vi "ListSelectedValue.vi"(8 "Language":u32, 9 "值表数组":string[][](array[string]), 10 "已选信号列表":string[][](array[string])) -> (3 "SelectList":string(tree))   [LabVIEW 2015]
panel:
  out "txtTitle":string
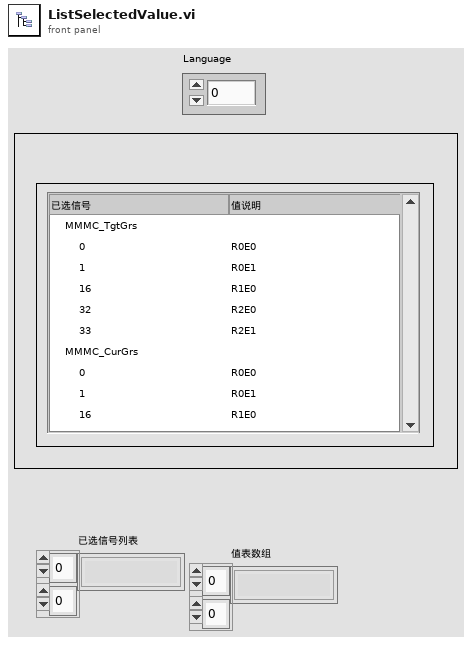
[diagram p1: front panel]
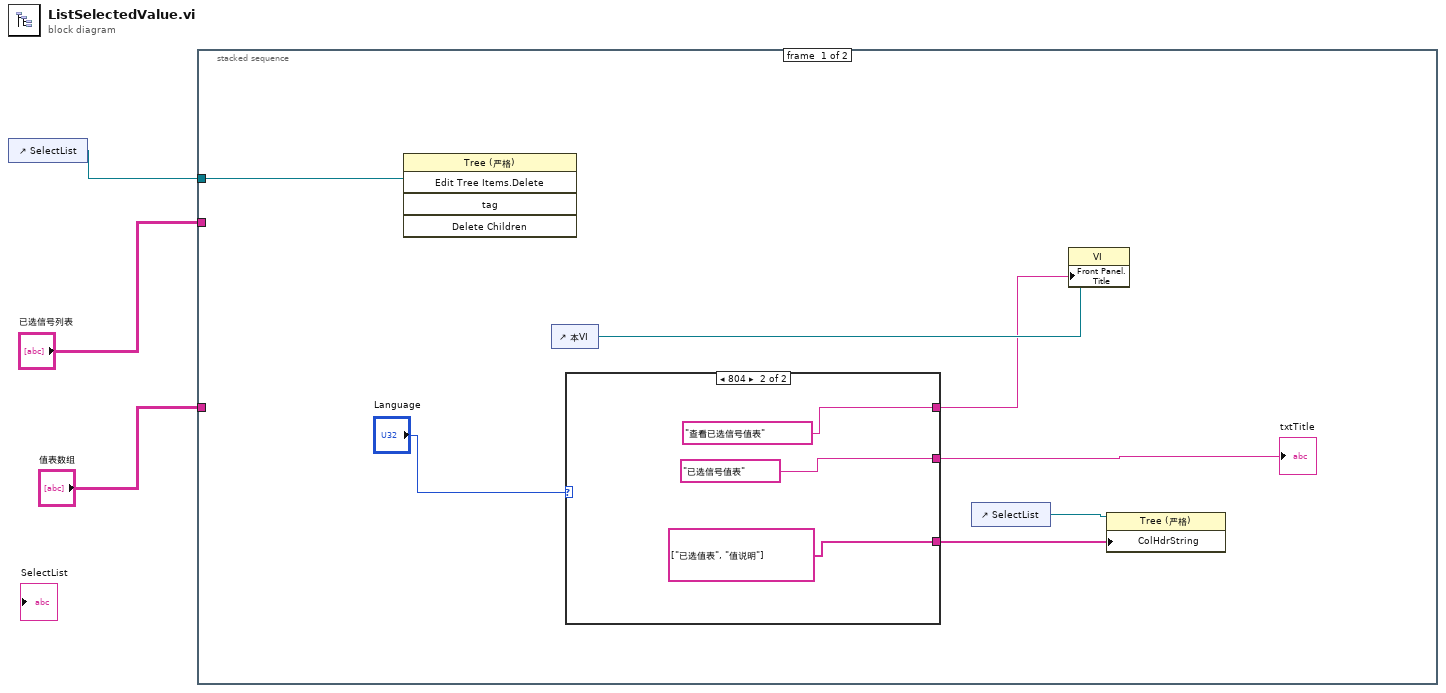
[diagram p0: block diagram]
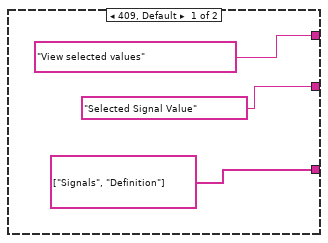
[diagram p2: hidden frame]
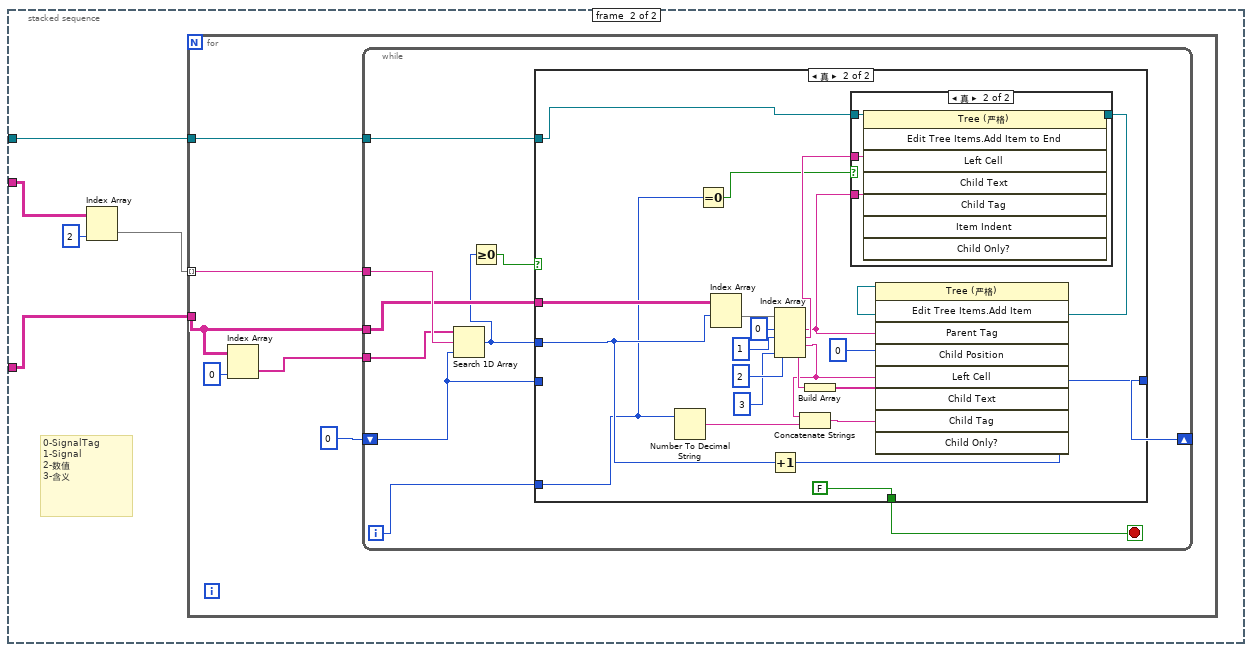
[diagram p3: hidden frame]
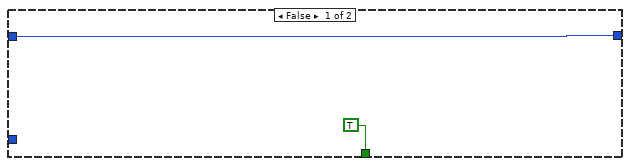
[diagram p4: hidden frame]
diagram:
  n1 = control-ref of="SelectList"() -> (w3:refnum<vi>)
  n2 = stacked-sequence {
    tunnel: w3 -> [w10 w19]
    tunnel: "值表数组" -> [_ w18]
    tunnel: "已选信号列表" -> [_ w17]
    frame #0 {
      n3 = invoke class="Tree (严格)" method="Edit Tree Items.Delete"(reference=w10) -> ()  [unwired: 4 in, 5 out]
      n4 = control-ref of="本VI"() -> (w8:refnum<vi>)
      n5 = case shown="804" "Language" {
        tunnel: ["View selected values" "查看已选信号值表"] -> w7
        tunnel: [string[] ["Signals", "Definition"] string[] ["已选值表", "值说明"]] -> w5
        tunnel: ["Selected Signal Value" "已选信号值表"] -> w4
        frame 409, Default {
        }
        frame 804 {
        }
      }
      "txtTitle" <- w4
      n6 = control-ref of="SelectList"() -> (w6:refnum<vi>)
      n7 = property class="VI"(reference=w8, "Front Panel.Title"=w7) -> ()  [unwired: 1 in, 2 out]
      n8 = property class="Tree (严格)"(reference=w6, "ColHdrString"=w5) -> ()  [unwired: 1 in, 2 out]
    }
    frame #1 {
      # "0-SignalTag\n1-Signal\n2-数值\n3-含义"
      n9 = Index Array(array=w17, index (col)=2 ("禁用的索引 (列)")) -> (element=w21:string[])  [unwired: 1 in]
      n10 = for {
        tunnel: w21 -> [w27] mode=indexing
        tunnel: w18 -> [w22]
        tunnel: w19 -> [w26]
        n11 = Index Array(array=w22, index (col)=0 ("禁用的索引 (列)")) -> (element=w23:string[])  [unwired: 1 in]
        n12 = while {
          tunnel: w27 -> [w37]
          tunnel: w22 -> [w36]
          tunnel: w26 -> [w35]
          shift-right: [w31] -> _
          shift-left: 0 -> [w30]
          tunnel: w23 -> [w28]
          i -> [w32]
          stop <- w29 stop-if-true
          n13 = Search 1D Array(1D array=w28, element=w37, start index (0)=w30) -> (index of element=w34:i32)
          n14 = Greater Or Equal To 0?(x=w34) -> (x >= 0?=w33:bool)
          n15 = case shown="真" w33 {
            tunnel: w36 -> [_ w60]
            tunnel: w35 -> [_ w42]
            tunnel: w32 -> [_ w41]
            tunnel: w34 -> [_ w47]
            tunnel: [w39 w46] -> w31
            tunnel: w30 -> [w39 _]
            tunnel: [TRUE FALSE] -> w29
            frame False {
            }
            frame True {
              n16 = Number To Decimal String(number=w41) -> (decimal integer string=w59:string)  [unwired: 1 in]
              n17 = Equal To 0?(x=w41) -> (x = 0?=w40:bool)
              n18 = Index Array(array=w60, index (row)=w47) -> (element=w58:string[])  [unwired: 1 in]
              n19 = Increment(x=w47) -> (x+1=w46:i32)
              n20 = Index Array(array=w58, index #1=0 ("索引"), index #2=1 ("索引"), index #3=2 ("索引"), index #4=3 ("索引")) -> (element #1=w44:string, element #2=w53:string, element #3=w49:string, element #4=w50:string)
              n21 = Concatenate Strings(w49, w59) -> (w48:string)
              n22 = Build Array(w50) -> (w51:string[])
              n23 = case shown="真" w40 {
                tunnel: w53 -> [_ w65]
                tunnel: w42 -> [w61 w64]
                tunnel: w44 -> [_ w63]
                tunnel: [w61 w62] -> w43
                frame False {
                }
                frame True {
                  n24 = invoke class="Tree (严格)" method="Edit Tree Items.Add Item to End"(reference=w64, "Left Cell"=w65, "Child Tag"=w63) -> (reference out=w62:refnum<vi>)  [unwired: 5 in, 7 out]
                }
              }
              n25 = invoke class="Tree (严格)" method="Edit Tree Items.Add Item"(reference=w43, "Parent Tag"=w44, "Child Position"=0 ("子项位置"), "Left Cell"=w49, "Child Text"=w51, "Child Tag"=w48) -> ()  [unwired: 3 in, 9 out]
            }
          }
        }
      }
    }
  }
